vi "Array Point to RowCol V3.vi"(8 "error in (no error)":errorcluster, 10 "PID":refnum<vi>, 11 "top array":refnum<vi>) -> (0 "error out":errorcluster, 1 "Flatline?":bool, 2 "Index":i32, 3 "PID key focus?":bool)   [LabVIEW 2021, in "RocketPlot.lvlib"]
uses:
  RocketPlot.lvlib
  TypeDefs/Plot top row.ctl
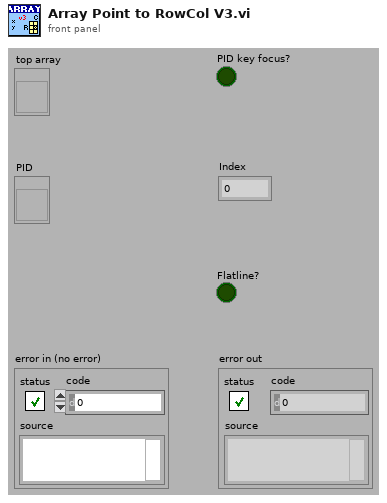
[diagram p1: front panel]
types:
  T1 = typedef "RocketPlot.lvlib/Plot top row.ctl" = cluster{"PID":string, "index":i32, "PID color":u32, "right axis?":bool, "Flatline?":bool, "Numeric color":u32, "Data":string, "Flat":string}
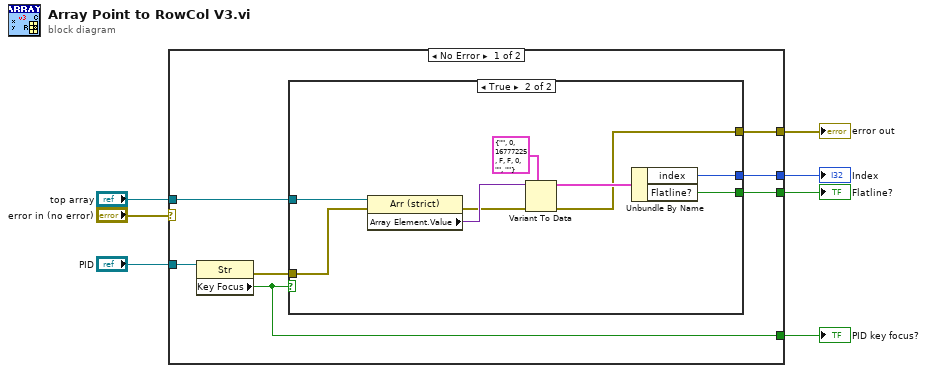
[diagram p0: block diagram]
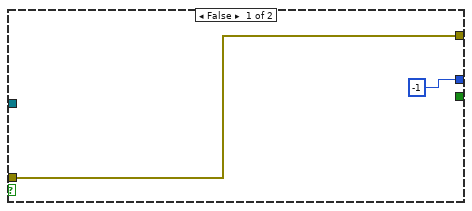
[diagram p2: hidden frame]
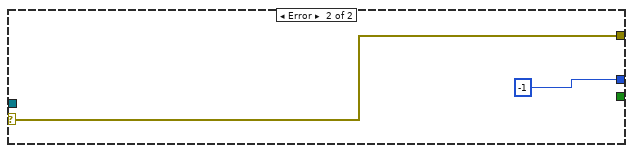
[diagram p3: hidden frame]
diagram:
  n1 = case shown="No Error" "error in (no error)" {
    selector: "error in (no error)" -> [_ w27]
    tunnel: "top array" -> [w14 _]
    tunnel: [w13 w27] -> w6
    tunnel: [w10 _] -> w5
    tunnel: "PID" -> [w12 _]
    tunnel: [w9 -1 ("index")] -> w3
    tunnel: [w8 _] -> w2
    frame No Error {
      n2 = property class="Str"(reference=w12) -> (error out=w11:errorcluster, "Key Focus"=w10:bool)  [unwired: 1 in, 1 out]
      n3 = case shown="True" w10 {
        tunnel: w14 -> [_ w25]
        tunnel: [w16 w18] -> w13
        tunnel: w11 -> [w16 w24]
        tunnel: [-1 ("Index") w20] -> w9
        tunnel: [_ w17] -> w8
        frame False {
        }
        frame True {
          n4 = property class="Arr (strict)"(reference=w25, error in=w24) -> (error out=w19:errorcluster, "Array Element.Value"=w22:variant)  [unwired: 1 out]
          n5 = Variant To Data(error in=w19, type=T1 {"PID"="", "index"=0, "PID color"=16777225, "right axis?"=FALSE, "Flatline?"=FALSE, "Numeric color"=0, "Data"="", "Flat"=""} ("Cluster 2"), Variant=w22) -> (data=w21:T1, error out=w18:errorcluster)
          n6 = Unbundle By Name(w21) -> ("index"=w20:i32, "Flatline?"=w17:bool)
        }
      }
    }
    frame Error {
    }
  }
  "error out" <- w6
  "Index" <- w3
  "PID key focus?" <- w5
  "Flatline?" <- w2
